vi "Redis@GetRecord__Parameter.vi"(1 "ParamterIn":string) -> (0 "ParamterOut":string)   [LabVIEW 2020]
panel:
  in  "LastOne=":string(combo)
  in  "Dir=":string(combo)
  in  "Message=":string
  in  "TimeOut=":string(combo)
  in  "Variable=":string(combo)
  in  "Section":string(combo)
  in  "CMD":string
  in  "RedisSession":string(combo)
  in  "Confirm":bool
  # "RedisSession(,Variable=,TimeOut=XXX, Message=XXX,LastOne={0,1} )"
  # "@"
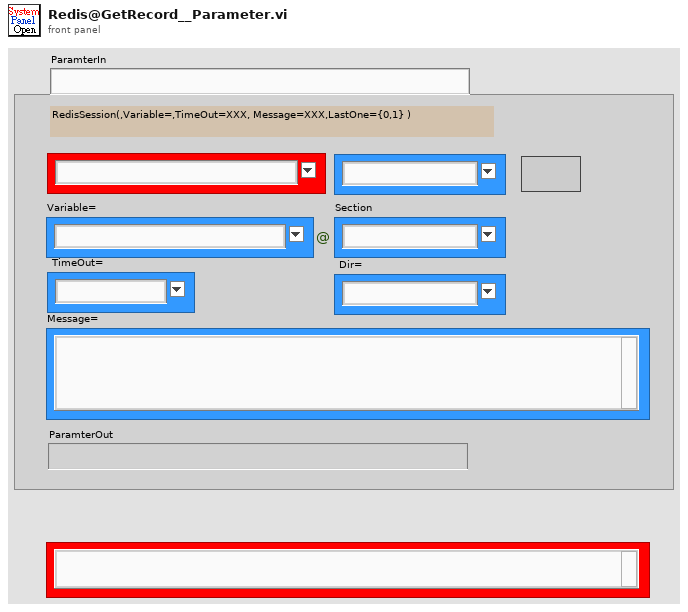
[diagram p1: front panel]
types:
  T1 = enum16{"Get", "Init", "Set", "Delete", "GetElement", "Inc", "Dec"}
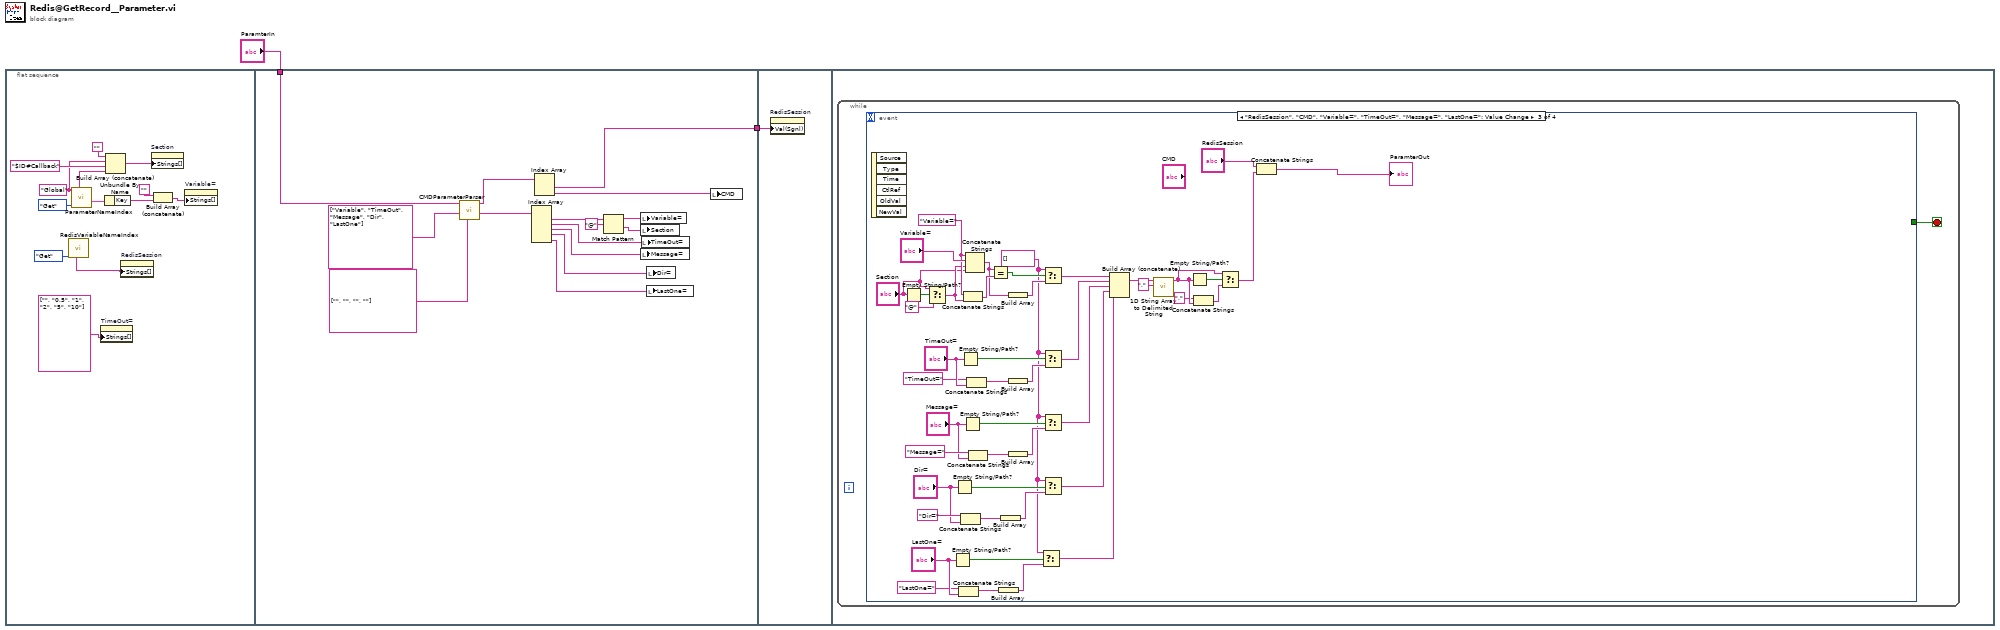
[diagram p0: block diagram]
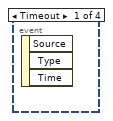
[diagram p2: hidden frame]
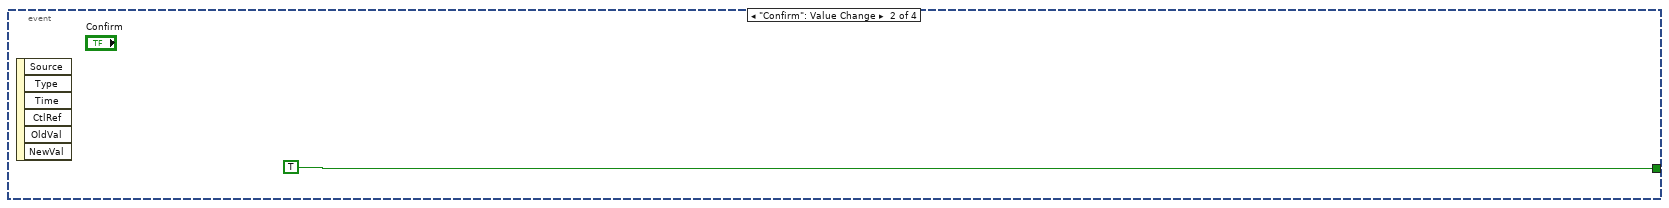
[diagram p3: hidden frame]
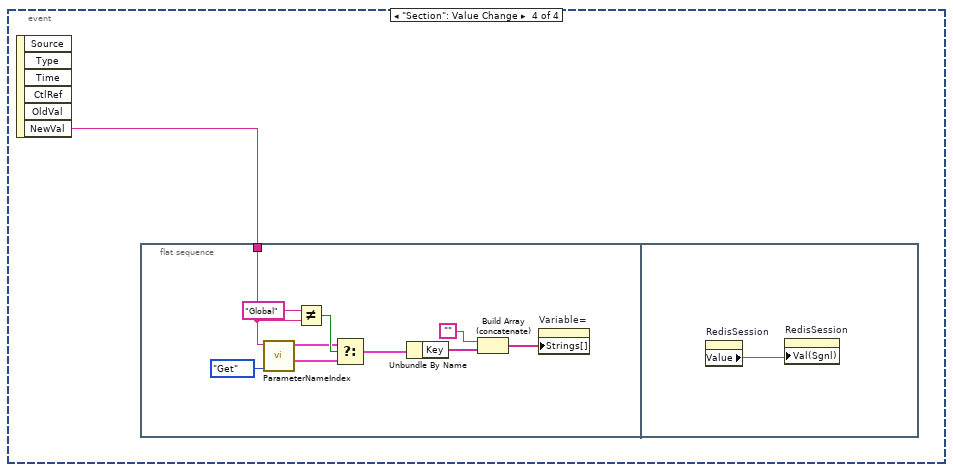
[diagram p4: hidden frame]
diagram:
  n1 = flat-sequence {
    tunnel: "ParamterIn" -> [w30]
    tunnel: [w26] -> w1
    tunnel: w1 -> [w31]
    frame #0 {
      w6 = "Global" ("VariableSection")
      n2 = call "RedisVariableNameIndex.vi"("OP"=enum16{"Add", "Init", "Get"}."Get") -> ("RedisSessionS"=w8:string[])  [unwired: 6 in, 4 out]
      n3 = call "ParameterNameIndex.vi"("OP"=T1."Get", "VariableSection"=w6) -> ("GlobalKeyValue"=w7:cluster{"Key":string[], "Value":string[]}, "SectionList"=w14:string[])  [unwired: 3 in, 5 out]
      n4 = property on="TimeOut=" class="CmbBox"("Strings[]"=string[] ["", "0.5", "1", "2", "5", "10"] ("Strings []")) -> ()  [unwired: 2 in, 2 out]
      n5 = Unbundle By Name(w7) -> ("Key"=w4:string[])
      n6 = Build Array (concatenate)("", w6, "$ID#Callback" ("VariableSection"), w14) -> (w13:string[])
      n7 = property on="RedisSession" class="CmbBox"("Strings[]"=w8) -> ()  [unwired: 2 in, 2 out]
      n8 = property on="Section" class="CmbBox"("Strings[]"=w13) -> ()  [unwired: 2 in, 2 out]
      n9 = Build Array (concatenate)("", w4) -> (w3:string[])
      n10 = property on="Variable=" class="CmbBox"("Strings[]"=w3) -> ()  [unwired: 2 in, 2 out]
    }
    frame #1 {
      n11 = call "CMDParameterParser.vi"("DeafultValues"=string[] ["", "", "", ""], "RequiredKeys"=string[] ["Variable", "TimeOut", "Message", "Dir", "LastOne"], "CMDParameter"=w30) -> ("KeyValues"=w24:string[], "Input"=w27:string[])  [unwired: 6 in, 1 out]
      n12 = Index Array(array=w24) -> (element #1=w23:string, element #2=w20:string, element #3=w19:string, element #4=w17:string, element #5=w16:string)  [unwired: 5 in]
      n13 = Index Array(array=w27) -> (element #1=w26:string, element #2=w25:string)  [unwired: 2 in]
      n14 = Match Pattern(string=w23, regular expression="@") -> (before substring=w21:string, after substring=w18:string)  [unwired: 1 in, 2 out]
      n15 = local write "Variable="(w21) -> ()
      n16 = local write "Section"(w18) -> ()
      n17 = local write "Message="(w19) -> ()
      n18 = local write "TimeOut="(w20) -> ()
      n19 = local write "Dir="(w17) -> ()
      n20 = local write "LastOne="(w16) -> ()
      n21 = local write "CMD"(w25) -> ()
    }
    frame #2 {
      n22 = property on="RedisSession" class="CmbBox"("Val(Sgnl)"=w31) -> ()  [unwired: 2 in, 2 out]
    }
    frame #3 {
      n23 = while {
        stop <- w32 stop-if-true
        n24 = event shown="[2] \"RedisSession\", \"CMD\", \"Variable=\", \"TimeOut=\", \"Message=\", \"LastOne=\": Value Change" {
          selector: _ -> [_ _ _ _]
          dyn-events: _ -> [_ _ _ _]
          timeout: _ -> [_ _ _ _]
          tunnel: [_ TRUE _ _] -> w32
          event Timeout {
            n25 = event-data() -> ()  [unwired: 1 in, 3 out]
          }
          event "Confirm": Value Change {
            n26 = event-data() -> ()  [unwired: 1 in, 6 out]
          }
          event "RedisSession", "CMD", "Variable=", "TimeOut=", "Message=", "LastOne=": Value Change {
            w36 = string[] [] ("t")
            w74 = "Variable=" ("string")
            n27 = event-data() -> ()  [unwired: 1 in, 6 out]
            n28 = Empty String/Path?(string/path="Section") -> (empty?=w51:bool)
            n29 = Select(t="Section", s=w51, f="@") -> (s? t:f=w49:string)
            n30 = Empty String/Path?(string/path="LastOne=") -> (empty?=w39:bool)
            n31 = Empty String/Path?(string/path="Dir=") -> (empty?=w45:bool)
            n32 = Concatenate Strings("LastOne=" ("string"), "LastOne=") -> (w38:string)
            n33 = Empty String/Path?(string/path="TimeOut=") -> (empty?=w73:bool)
            n34 = Concatenate Strings("Dir=" ("string"), "Dir=") -> (w46:string)
            n35 = Empty String/Path?(string/path="Message=") -> (empty?=w68:bool)
            n36 = Concatenate Strings(w74, w49) -> (w67:string)
            n37 = Concatenate Strings(w74, "Variable=", w49, "Section") -> (w52:string)
            n38 = Concatenate Strings("TimeOut=" ("string"), "TimeOut=") -> (w65:string)
            n39 = Concatenate Strings("Message=" ("string"), "Message=") -> (w63:string)
            n40 = Equal?(x=w52, y=w67) -> (x = y?=w75:bool)
            n41 = Build Array(w38) -> (w37:string[])
            n42 = Build Array(w46) -> (w47:string[])
            n43 = Build Array(w52) -> (w66:string[])
            n44 = Build Array(w65) -> (w64:string[])
            n45 = Build Array(w63) -> (w62:string[])
            n46 = Select(t=w36, s=w39, f=w37) -> (s? t:f=w35:string[])
            n47 = Select(t=w36, s=w75, f=w66) -> (s? t:f=w61:string[])
            n48 = Select(t=w36, s=w73, f=w64) -> (s? t:f=w60:string[])
            n49 = Select(t=w36, s=w68, f=w62) -> (s? t:f=w59:string[])
            n50 = Select(t=w36, s=w45, f=w47) -> (s? t:f=w43:string[])
            n51 = Build Array (concatenate)(w61, w60, w59, w43, w35) -> (w58:string[])
            n52 = call <vilib>:"1D String Array to Delimited String.vi"("delimiter"=",", "string array"=w58) -> ("delimited string"=w55:string)  [unwired: 9 in]
            n53 = Empty String/Path?(string/path=w55) -> (empty?=w56:bool)
            n54 = Concatenate Strings("," ("string"), w55) -> (w53:string)
            n55 = Select(t=w55, s=w56, f=w53) -> (s? t:f=w34:string)
            n56 = Concatenate Strings("RedisSession", w34) -> (→"ParamterOut":string)
          }
          event "Section": Value Change {
            n57 = event-data() -> ("NewVal"=w79:string)  [unwired: 1 in, 5 out]
            n58 = flat-sequence {
              tunnel: w79 -> [w88]
              frame #0 {
                n59 = call "ParameterNameIndex.vi"("OP"=T1."Get", "VariableSection"=w88) -> ("GlobalKeyValue"=w84:cluster{"Key":string[], "Value":string[]}, "SectionKeyValue"=w85:cluster{"Key":string[], "Value":string[]})  [unwired: 3 in, 5 out]
                n60 = Not Equal?(x="Global", y=w88) -> (x != y?=w86:bool)
                n61 = Select(t=w85, s=w86, f=w84) -> (s? t:f=w83:cluster{"Key":string[], "Value":string[]})
                n62 = Unbundle By Name(w83) -> ("Key"=w82:string[])
                n63 = Build Array (concatenate)("", w82) -> (w80:string[])
                n64 = property on="Variable=" class="CmbBox"("Strings[]"=w80) -> ()  [unwired: 2 in, 2 out]
              }
              frame #1 {
                n65 = property on="RedisSession" class="CmbBox"() -> ("Value"=w90:string)  [unwired: 2 in, 2 out]
                n66 = property on="RedisSession" class="CmbBox"("Val(Sgnl)"=w90) -> ()  [unwired: 2 in, 2 out]
              }
            }
          }
        }
      }
    }
  }
